vi "acquire multi waves.vi"() -> ()   [LabVIEW 2013]
panel:
  out "CH2 VOLTS/DIV":string
  out "CH1 VOLTS/DIV":string
  out "Waveform Graph":i32[][](graph)
  out "CH2 PROBE":string
  out "CH2 SCALE":string
  out "CH2":string
  in  "stop":bool
  in  "VISA resource name":refnum<visa-resource-name>="USB0::0x5345::0x1234::SERIAL::RAW"
  out "SEC/DIV":string
  out "CH1":string
  out "CH1 PROBE":string
  out "CH1":string
  # "1.Fill in the visa resource name of your device"
  # "2.Please use the stop button to stop the vi"
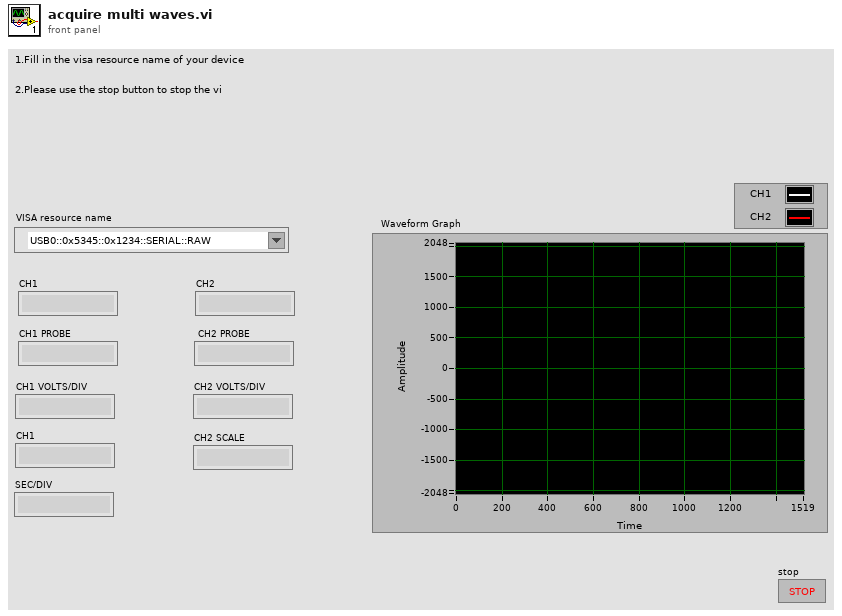
[diagram p1: front panel]
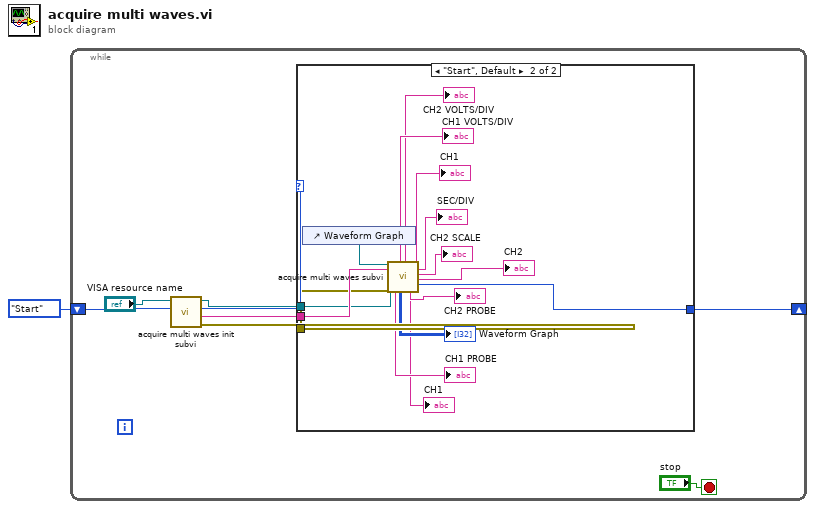
[diagram p0: block diagram]
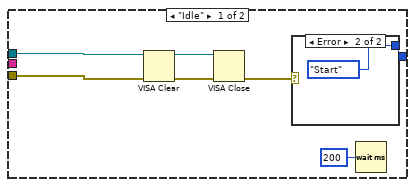
[diagram p2: hidden frame]
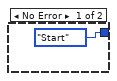
[diagram p3: hidden frame]
diagram:
  n1 = while {
    shift-right: [w4] -> _
    shift-left: enum16{"Idle", "Start"}."Start" -> [w6]
    stop <- "stop" stop-if-true
    n2 = call "acquire multi waves init subvi.vi"("Enum in"=w6, "VISA Refnum in"="VISA resource name") -> ("error out"=w8:errorcluster, "read buffer"=w7:string, "Enum out"=w5:enum16{"Idle", "Start"}, "VISA Refnum out"=w9:refnum<visa-resource-name>)  [unwired: 6 in]
    n3 = case shown="\"Start\", Default" w5 {
      tunnel: w9 -> [w13 w31]
      tunnel: w8 -> [w12 w30]
      tunnel: w7 -> [_ w33]
      tunnel: [w16 w32] -> w4
      frame "Idle" {
        n4 = VISA Clear(VISA resource name=w13, error in (no error)=w12) -> (VISA resource name out=w15:refnum<visa-resource-name>, error out=w14:errorcluster)
        n5 = VISA Close(VISA resource name=w15, error in (no error)=w14) -> (error out=w11:errorcluster)
        n6 = case shown="Error" w11 {
          tunnel: [enum16{"Idle", "Start"}."Start" enum16{"Idle", "Start"}."Start"] -> w16
          frame No Error {
          }
          frame Error {
          }
        }
        n7 = Wait (ms)(milliseconds to wait=u32 200 ("等待时间（毫秒）")) -> ()  [unwired: 1 out]
      }
      frame "Start", Default {
        n8 = control-ref of="Waveform Graph"() -> (w28:refnum<vi>)
        n9 = call "acquire multi waves subvi.vi"("WaveformGraph in"=w28, "read buffer"=w33, "VISA Refnum in"=w31, "error in (no error)"=w30) -> ("CH1 PROBE"=→"CH1 PROBE":string, "CH1 VOLTS/DIV"=→"CH1 VOLTS/DIV":string, "Array"=→"Waveform Graph":i32[][], "CH2 VOLTS/DIV"=→"CH2 VOLTS/DIV":string, "CH1 2"=→"CH1":string, "CH2 PROBE"=→"CH2 PROBE":string, "CH1"=→"CH1":string, "SEC/DIV"=→"SEC/DIV":string, "CH2 SCALE"=→"CH2 SCALE":string, "CH2"=→"CH2":string, "Enum"=w32:enum16{"Idle", "Start"})  [unwired: 4 in, 1 out]
      }
    }
  }
